vi "Tenney Main.vi"() -> ()   [LabVIEW 2023]
doc: "This template is for the Queued Message Handler design pattern.\n\nThe Event Handling Loop generates messages based on user interface actions.\n\nThe Message Handling Loop processes messages generated by the Event Handling Loop, or by other messages. The messages are string values, so new messages can be added easily to the Message Cases case structure in the Message Handling Loop. Each message cluster can also provide an optional value for Message Data, which is a variant that can be converted to whatever message-specific data is required."
uses:
  Drivers/Tidal Engineering/Type Definitions/Tenney Environmental Chamber Data.ctl
  controls/Tenney Temperature Limits.ctl
  Drivers/Viasala Indigo 520/Type Definitions/Viasala Indigo 520 Data.ctl
  Drivers/Tidal Engineering/Type Definitions/Tenney Chamber Status.ctl
  controls/Tenney UI Data.ctl
  support/Message Queue/Enqueue Message (Single).vi
  <vilib>/Utility/error.llb/Error Cluster From Error Code.vi
  <vilib>/ErrorRing/Error Ring.xnode
  support/Message Queue/Tenney Message Queue.lvlib
  support/User Event - Stop/Tenney User Event - Stop.lvlib
panel:
  in  "Tab Control":enum32{"Main", "Admin", "Debug Array"}(tab)
  in  "Chamber Status":T1
  in  "Set Status":bool
  in  "Set Temperature":bool
  in  "Set Humidity":bool
  in  "Set Frequency":bool
  in  "Setpoint Temperature (F)":dbl=67.5 min=32.0 max=135.0
  in  "Setpoint Humidity (%)":dbl=50.0 min=0.0 max=100.0
  in  "Setpoint Frequency (Hz)":dbl=10.0 min=5.0 max=60.0
  in  "Temperature Limits":T2={"Target Temperature Upper limit"=68.75, "Target Temperature Lower limit"=67.75, "Target Humidity Lower limit"=48.5, "Target Humidity Upper limit"=50.5, "Chamber Temperature Upper limit"=73.0, "Chamber Temperature Lower limit"=63.0, "Chamber Humidity Lower limit"=40.0, "Chamber Humidity Upper limit"=55.0, "Chamber Adjustment Increment (F)"=0.25, "Chamber Adjustment Interval (Minutes)"=10.0, "Chamber Adjustment Increment (%)"=0.25, "Chamber Adjustment Interval Fast (Minutes)"=10.0}
  in  "Update Temperature Limits":bool
  out "Tenney Data":T3
  out "Viasala Data Output":T4
  in  "Elapsed Time (Min)":dbl
  in  "Enable Auto Control":bool
  in  "Sample Rate (mS)":u32=10000
  in  "Viasala Loop Counter":i32
  in  "Viasala IP Address":string="10.2.0.39"
  in  "Tenney IP Address":string="10.2.0.248"
  in  "Debug":bool
  in  "Tenney Chamber Loop Counter":i32
  in  "Data Array":dbl[][](array[numeric])
  in  "Connect Viasala Counter":dbl
  in  "Connect Tenney Counter":dbl
  out "Main Array":string[](array[string])
  out "Tenney Array":string[](array[string])
  out "Viasala Array":string[](array[string])
  in  "Enable Arrays":bool
  in  "Exit":bool
  # "Tenney Chamber Manual Control"
  # "Data Output"
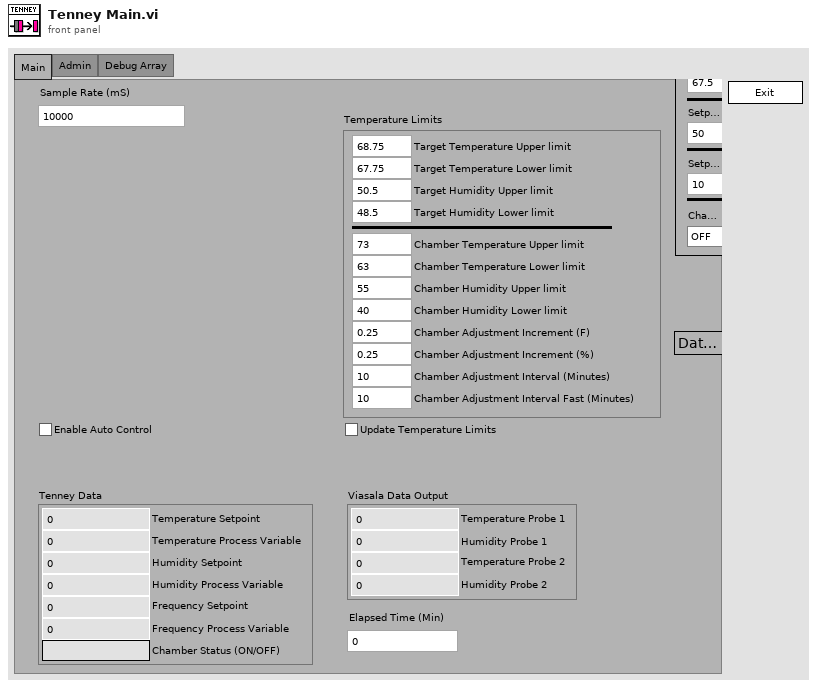
[diagram p1: front panel]
types:
  T1 = typedef "Tenney Chamber Status.ctl" = enum16{"OFF", "ON"}
  T2 = typedef "Tenney Temperature Limits.ctl" = cluster{"Target Temperature Upper limit":dbl, "Target Temperature Lower limit":dbl, "Target Humidity Lower limit":dbl, "Target Humidity Upper limit":dbl, "Chamber Temperature Upper limit":dbl, "Chamber Temperature Lower limit":dbl, "Chamber Humidity Lower limit":dbl, "Chamber Humidity Upper limit":dbl, "Chamber Adjustment Increment (F)":dbl, "Chamber Adjustment Interval (Minutes)":dbl, "Chamber Adjustment Increment (%)":dbl, "Chamber Adjustment Interval Fast (Minutes)":dbl}
  T3 = typedef "Tenney Environmental Chamber Data.ctl" = cluster{"Temperature Setpoint":dbl, "Temperature Process Variable":dbl, "Humidity Setpoint":dbl, "Humidity Process Variable":dbl, "Frequency Setpoint":dbl, "Frequency Process Variable":dbl, "Chamber Status (ON/OFF)":string}
  T4 = typedef "Viasala Indigo 520 Data.ctl" = cluster{"Temperature Probe 1":dbl, "Humidity Probe 1":dbl, "Temperature Probe 2":dbl, "Humidity Probe 2":dbl}
  T5 = typedef "Tenney UI Data.ctl" = cluster{"User Message":string, "Do Something Ref":refnum<vi>, "Do Something Else Ref":refnum<vi>, "Exit Button Ref":refnum<vi>}
  T6 = typedef "Tenney Message Queue.lvlib/All Message Queues.ctl" = cluster{"UI":refnum<queue>, "Tenney Chamber":refnum<queue>, "Viasala Humidity":refnum<queue>}
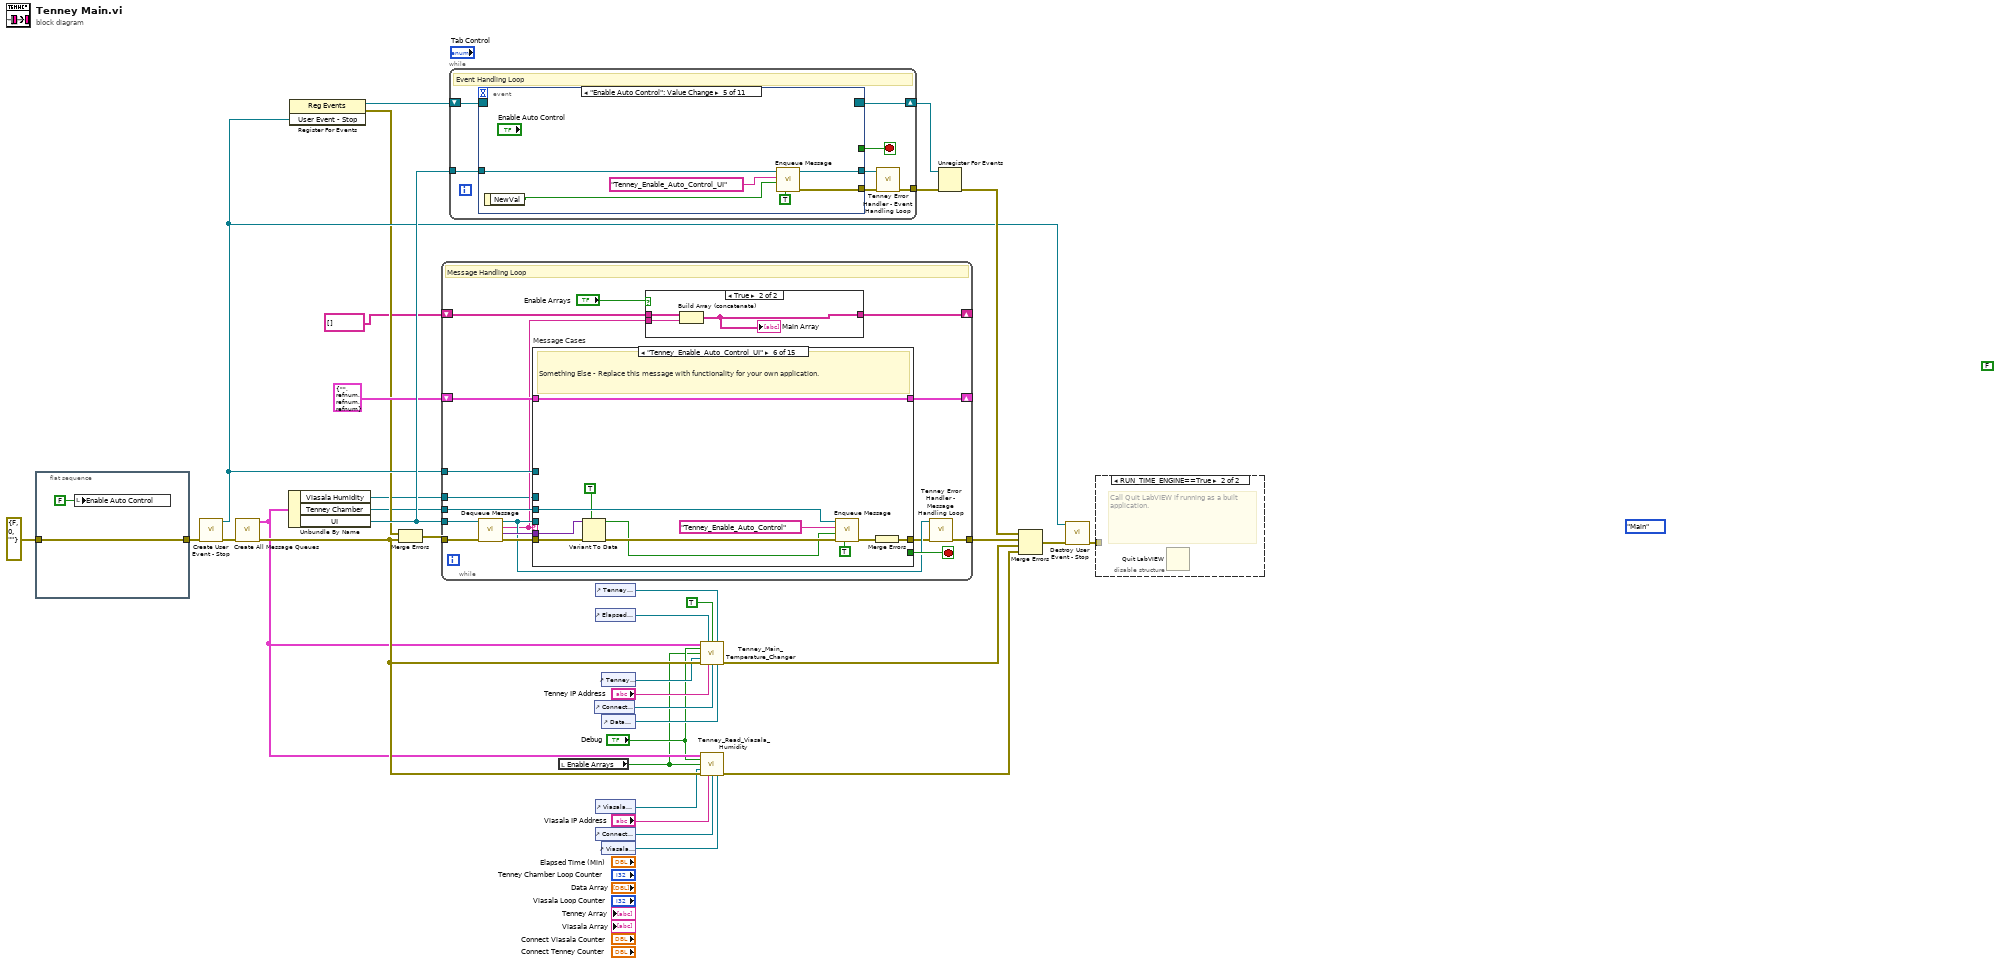
[diagram p0: block diagram]
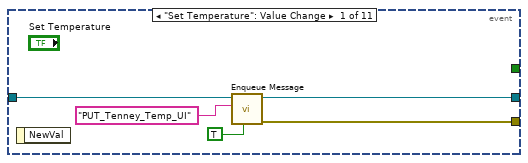
[diagram p3: hidden frame]
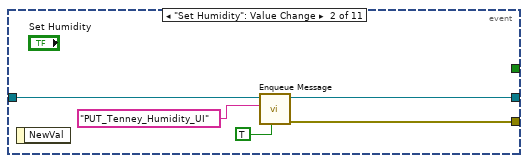
[diagram p4: hidden frame]
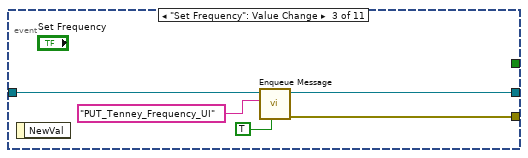
[diagram p5: hidden frame]
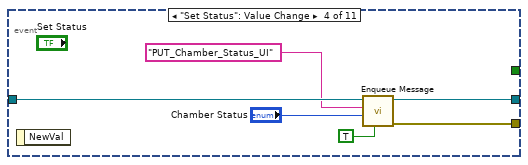
[diagram p6: hidden frame]
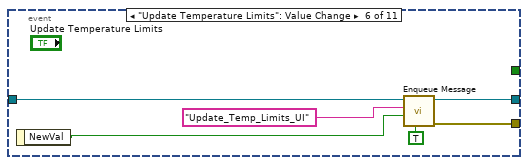
[diagram p7: hidden frame]
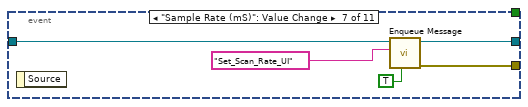
[diagram p8: hidden frame]
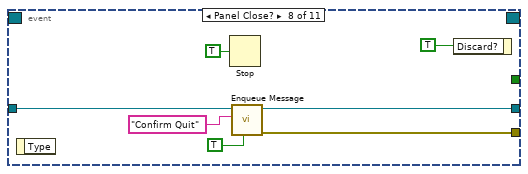
[diagram p9: hidden frame]
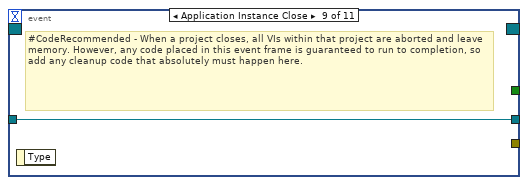
[diagram p10: hidden frame]
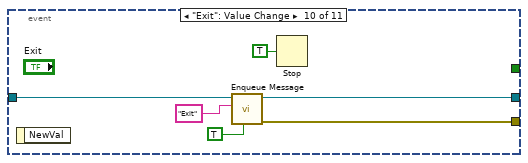
[diagram p11: hidden frame]
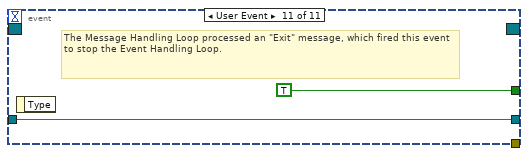
[diagram p12: hidden frame]
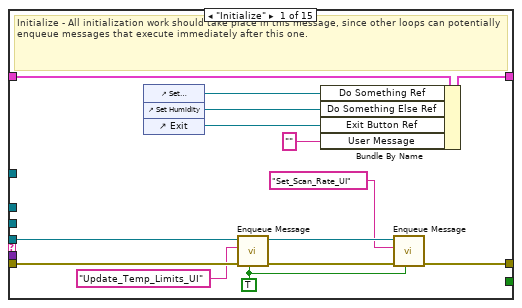
[diagram p14: hidden frame]
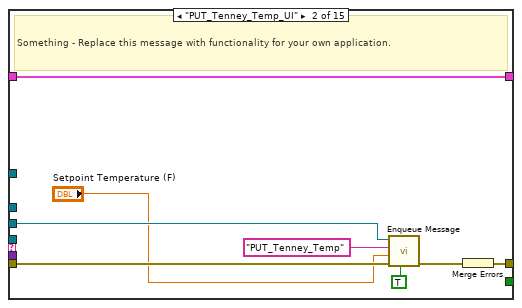
[diagram p15: hidden frame]
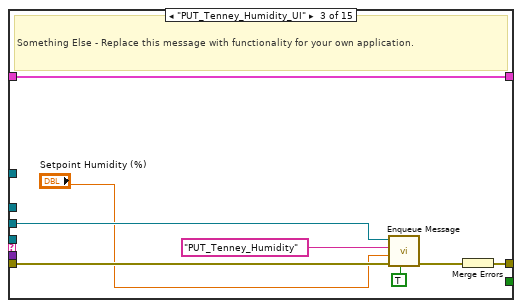
[diagram p16: hidden frame]
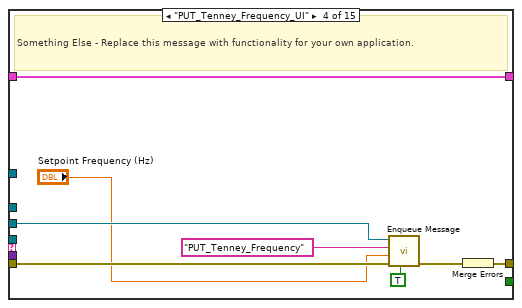
[diagram p17: hidden frame]
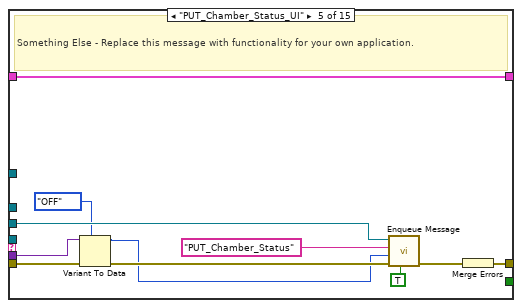
[diagram p18: hidden frame]
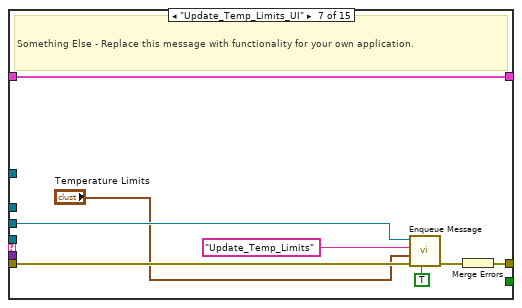
[diagram p19: hidden frame]
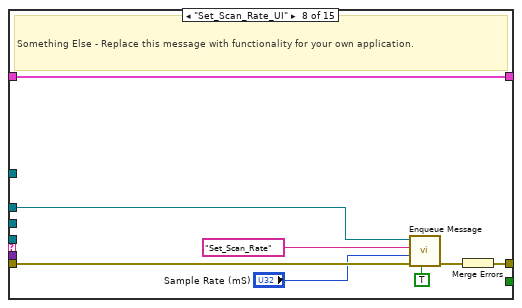
[diagram p20: hidden frame]
diagram:
  (unwired) FALSE ("Exit")
  (unwired) enum32{"Main", "Admin", "Debug Array"}."Main" ("Tab Control 8")
  n1 = flat-sequence {
    tunnel: errorcluster {"status"=FALSE, "code"=0, "source"=""} ("error in (no error)") -> [w37]
    tunnel: [w37] -> w18
    frame #0 {
      n2 = local write "Enable Auto Control"(FALSE ("Enable Auto Control")) -> ()
    }
  }
  n3 = call "Create User Event - Stop.vi"("error in (no error)"=w18) -> ("error out"=w33:errorcluster, "User Event - Stop"=w25:refnum<user-event>)  [unwired: 9 in]
  n4 = call "Create All Message Queues.vi"("error in (no error)"=w33) -> ("error out"=w17:errorcluster, "Message Queues out"=w15:T6)  [unwired: 9 in]
  n5 = Unbundle By Name(w15) -> ("Viasala Humidity"=w12:refnum<queue>, "Tenney Chamber"=w21:refnum<queue>, "UI"=w34:refnum<queue>)
  n6 = register-events(w25) -> (reference out=w26:refnum<event-registration>, error out=w23:errorcluster)  [unwired: 2 in]
  n7 = Merge Errors(w23, w17) -> (w24:errorcluster)
  n8 = while {
    tunnel: w34 -> [w47]
    shift-right: [w53] -> _
    shift-left: T5 {"User Message"="", "Do Something Ref"=refnum, "Do Something Else Ref"=refnum, "Exit Button Ref"=refnum} ("Data Cluster") -> [w54]
    tunnel: w25 -> [w51]
    tunnel: w24 -> [w50]
    tunnel: [w45] -> w35
    tunnel: w21 -> [w43]
    shift-right: [w41] -> _
    shift-left: string[] [] -> [w42]
    tunnel: w12 -> [w39]
    stop <- w52 stop-if-true
    # "Message Handling Loop"
    n9 = call "Dequeue Message.vi"("error in (no error)"=w50, "Message Queue"=w47) -> ("error out"=w49:errorcluster, "Message Data"=w48:variant, "Message"=w40:string, "dup Message Queue"=w46:refnum<queue>)  [unwired: 6 in]
    n10 = case "Message Cases" shown="\"Tenney_Enable_Auto_Control_UI\"" w40 {
      selector: w40 -> [_ _ _ _ _ _ _ _ _ _ _ _ _ _ w183]
      tunnel: w46 -> [w66 _ _ _ _ _ _ _ _ _ _ w158 _ w182 _]
      tunnel: w49 -> [w65 w78 w86 w94 w101 w112 w120 w129 w139 w146 w155 w162 w165 w176 _]
      tunnel: [w62 w79 w87 w95 w106 w117 w125 w133 w140 w147 w149 w160 w163 w179 w184] -> w44
      tunnel: w54 -> [w72 w80 w88 w96 w107 w118 w126 w134 w141 w148 w154 w161 w164 w181 w185]
      tunnel: [w71 w80 w88 w96 w107 w118 w126 w134 w141 w148 w154 w161 w164 w181 w185] -> w53
      tunnel: [_ _ _ _ _ _ _ _ _ _ _ _ _ TRUE _] -> w52
      tunnel: w48 -> [_ _ _ _ w99 w110 _ _ w138 w145 w153 _ _ w173 _]
      tunnel: w51 -> [_ _ _ _ _ _ _ _ _ _ _ _ _ w178 _]
      tunnel: w43 -> [_ w75 w83 w91 w103 w114 w122 _ _ _ _ _ _ w171 _]
      tunnel: w39 -> [_ _ _ _ _ _ _ w127 _ _ _ _ _ w168 _]
      frame "Initialize" {
        w60 = TRUE ("Priority Message? (F)")
        # "Initialize - All initialization work should take place in this message, since other loops can potentially enqueue messages that execute immediately after this one."
        n11 = control-ref of="Set Temperature"() -> (w70:refnum<vi>)
        n12 = control-ref of="Set Humidity"() -> (w69:refnum<vi>)
        n13 = control-ref of="Exit"() -> (w68:refnum<vi>)
        n14 = call-poly "Enqueue Message.vi"("Priority Message? (F)"=w60, "error in (no error)"=w65, "Message"="Update_Temp_Limits_UI", "Message Queue"=w66) -> ("error out"=w63:errorcluster, "dup Message Queue"=w61:refnum<queue>)  [unwired: 6 in]
        n15 = Bundle By Name(cluster=w72, "Do Something Ref"=w70, "Do Something Else Ref"=w69, "Exit Button Ref"=w68, "User Message"="" ("Initial Message")) -> (w71:T5)
        n16 = call-poly "Enqueue Message.vi"("Priority Message? (F)"=w60, "error in (no error)"=w63, "Message"="Set_Scan_Rate_UI", "Message Queue"=w61) -> ("error out"=w62:errorcluster)  [unwired: 6 in, 1 out]
      }
      frame "PUT_Tenney_Temp_UI" {
        # "Something - Replace this message with functionality for your own application."
        n17 = call-poly "Enqueue Message.vi"("Priority Message? (F)"=TRUE, "error in (no error)"=w78, "Message Data"="Setpoint Temperature (F)", "Message"="PUT_Tenney_Temp", "Message Queue"=w75) -> ("error out"=w77:errorcluster)  [unwired: 5 in, 1 out]
        n18 = Merge Errors(w77) -> (w79:errorcluster)
      }
      frame "PUT_Tenney_Humidity_UI" {
        # "Something Else - Replace this message with functionality for your own application."
        n19 = call-poly "Enqueue Message.vi"("Priority Message? (F)"=TRUE, "error in (no error)"=w86, "Message Data"="Setpoint Humidity (%)", "Message"="PUT_Tenney_Humidity", "Message Queue"=w83) -> ("error out"=w85:errorcluster)  [unwired: 5 in, 1 out]
        n20 = Merge Errors(w85) -> (w87:errorcluster)
      }
      frame "PUT_Tenney_Frequency_UI" {
        # "Something Else - Replace this message with functionality for your own application."
        n21 = call-poly "Enqueue Message.vi"("Priority Message? (F)"=TRUE, "error in (no error)"=w94, "Message Data"="Setpoint Frequency (Hz)", "Message"="PUT_Tenney_Frequency", "Message Queue"=w91) -> ("error out"=w93:errorcluster)  [unwired: 5 in, 1 out]
        n22 = Merge Errors(w93) -> (w95:errorcluster)
      }
      frame "PUT_Chamber_Status_UI" {
        # "Something Else - Replace this message with functionality for your own application."
        n23 = Variant To Data(error in=w101, type=Tenney_Chamber_Status."OFF" ("Chamber Status"), Variant=w99) -> (data=w97:T1, error out=w100:errorcluster)
        n24 = call-poly "Enqueue Message.vi"("Priority Message? (F)"=TRUE, "error in (no error)"=w100, "Message Data"=w97, "Message"="PUT_Chamber_Status", "Message Queue"=w103) -> ("error out"=w105:errorcluster)  [unwired: 5 in, 1 out]
        n25 = Merge Errors(w105) -> (w106:errorcluster)
      }
      frame "Tenney_Enable_Auto_Control_UI" {
        # "Something Else - Replace this message with functionality for your own application."
        n26 = Variant To Data(error in=w112, type=TRUE, Variant=w110) -> (data=w109:bool, error out=w111:errorcluster)
        n27 = call-poly "Enqueue Message.vi"("Priority Message? (F)"=TRUE, "error in (no error)"=w111, "Message Data"=w109, "Message"="Tenney_Enable_Auto_Control", "Message Queue"=w114) -> ("error out"=w116:errorcluster)  [unwired: 5 in, 1 out]
        n28 = Merge Errors(w116) -> (w117:errorcluster)
      }
      frame "Update_Temp_Limits_UI" {
        # "Something Else - Replace this message with functionality for your own application."
        n29 = call-poly "Enqueue Message.vi"("Priority Message? (F)"=TRUE, "error in (no error)"=w120, "Message Data"="Temperature Limits", "Message"="Update_Temp_Limits", "Message Queue"=w122) -> ("error out"=w124:errorcluster)  [unwired: 5 in, 1 out]
        n30 = Merge Errors(w124) -> (w125:errorcluster)
      }
      frame "Set_Scan_Rate_UI" {
        # "Something Else - Replace this message with functionality for your own application."
        n31 = call-poly "Enqueue Message.vi"("Priority Message? (F)"=TRUE, "error in (no error)"=w129, "Message Data"="Sample Rate (mS)", "Message"="Set_Scan_Rate", "Message Queue"=w127) -> ("error out"=w132:errorcluster)  [unwired: 5 in, 1 out]
        n32 = Merge Errors(w132) -> (w133:errorcluster)
      }
      frame "DisplayValuesFromTenney" {
        # "Update Display - Convert the message data to a string to display in the Data Display indicator."
        n33 = Variant To Data(error in=w139, type=T3 {"Temperature Setpoint"=0.0, "Temperature Process Variable"=0.0, "Humidity Setpoint"=0.0, "Humidity Process Variable"=0.0, "Frequency Setpoint"=0.0, "Frequency Process Variable"=0.0, "Chamber Status (ON/OFF)"=""} ("Tenney Environmental Chamber Data"), Variant=w138) -> (data=→"Tenney Data":T3, error out=w137:errorcluster)
        n34 = Merge Errors(w137) -> (w140:errorcluster)
      }
      frame "DisplayValuesFromViasala" {
        # "Update Display - Convert the message data to a string to display in the Data Display indicator."
        n35 = Variant To Data(error in=w146, type=T4 {"Temperature Probe 1"=0.0, "Humidity Probe 1"=0.0, "Temperature Probe 2"=0.0, "Humidity Probe 2"=0.0} ("Viasala Data Output"), Variant=w145) -> (data=→"Viasala Data Output":T4, error out=w144:errorcluster)
        n36 = Merge Errors(w144) -> (w147:errorcluster)
      }
      frame "Error" {
        # "Error - Display an error dialog. This message is sent by the \"Error Handler\" VIs at the end of other loops in this application."
        n37 = Variant To Data(error in=w155, type=errorcluster {"status"=FALSE, "code"=0, "source"=""} ("error constant"), Variant=w153) -> (data=w151:errorcluster, error out=w150:errorcluster)
        n38 = call <vilib>:"Simple Error Handler.vi"("error in (no error)"=w151) -> ()  [unwired: 4 in, 5 out]
        n39 = Merge Errors(w150) -> (w149:errorcluster)
      }
      frame "Confirm Quit" {
        # "Confirm Quit - Message that can confirm whether or not the user wants to exit the application."
        n40 = call-poly "Enqueue Message.vi"("Priority Message? (F)"=TRUE, "error in (no error)"=w162, "Message"="Exit", "Message Queue"=w158) -> ("error out"=w159:errorcluster)  [unwired: 6 in, 1 out]
        n41 = Merge Errors(w159) -> (w160:errorcluster)
      }
      frame "---Copy This Frame---" {
        # "Duplicate this frame when creating new messages.  Change this comment in the duplicated frame to describe this message."
        n42 = Merge Errors(w165) -> (w163:errorcluster)
      }
      frame "Exit" {
        w166 = TRUE ("Priority Message? (F)")
        w167 = "Exit" ("Message")
        # "Exit - Exit the application."
        n43 = Variant To Data(type=errorcluster {"status"=FALSE, "code"=0, "source"=""} ("error constant"), Variant=w173) -> (data=w174:errorcluster)  [unwired: 1 in, 1 out]
        n44 = call <vilib>:"Simple Error Handler.vi"("error in (no error)"=w174) -> ()  [unwired: 4 in, 5 out]
        n45 = call "Fire User Event - Stop.vi"("User Event - Stop"=w178) -> ("error out"=w177:errorcluster)  [unwired: 10 in]
        n46 = Release Queue(queue=w182, error in (no error)=w176) -> (error out=w172:errorcluster)  [unwired: 1 in, 2 out]
        n47 = call-poly "Enqueue Message.vi"("Priority Message? (F)"=w166, "error in (no error)"=w172, "Message"=w167, "Message Queue"=w171) -> ("error out"=w170:errorcluster)  [unwired: 6 in, 1 out]
        n48 = call-poly "Enqueue Message.vi"("Priority Message? (F)"=w166, "error in (no error)"=w170, "Message"=w167, "Message Queue"=w168) -> ("error out"=w169:errorcluster)  [unwired: 6 in, 1 out]
        n49 = Merge Errors(w177, w169) -> (w179:errorcluster)
      }
      frame Default {
        # "'Default' case only runs if there is a message that isn't defined in any of the other cases.  Output a programming error."
        n50 = xnode "Error Ring"("parameter 0"=w183) -> ("error out"=w184:errorcluster)
      }
    }
    n51 = case shown="True" "Enable Arrays" {
      tunnel: w42 -> [w55 w58]
      tunnel: [w55 w57] -> w41
      tunnel: w40 -> [_ w56]
      frame False {
      }
      frame True {
        n52 = Build Array (concatenate)(w58, w56) -> (w57:string[])
        "Main Array" <- w57
      }
    }
    n53 = call "Tenney Error Handler - Message Handling Loop.vi"("error in (no error)"=w44, "Message Queue"=w46) -> ("dup error in"=w45:errorcluster)  [unwired: 8 in, 1 out]
  }
  n54 = while {
    tunnel: w34 -> [w199]
    shift-right: [w197] -> w30
    shift-left: w26 -> [w198]
    tunnel: [w193] -> w27
    stop <- w195 stop-if-true
    # "Event Handling Loop"
    n55 = event shown="[4] \"Enable Auto Control\": Value Change" {
      selector: w198 -> [_ _ _ _ _ _ _ _ _ _ _]
      dyn-events: [_ _ _ _ _ _ _ _ _ _ _] -> w197
      timeout: _ -> [_ _ _ _ _ _ _ _ _ _ _]
      tunnel: [_ _ _ _ _ _ _ _ _ _ TRUE ("Discard?")] -> w195
      tunnel: w199 -> [w204 w209 w214 w220 w226 w232 w235 w243 w245 w251 w253]
      tunnel: [w201 w206 w211 w217 w223 w229 w233 w242 _ w250 _] -> w196
      tunnel: [w203 w208 w213 w219 w225 w231 w234 w241 w245 w249 w253] -> w194
      event "Set Temperature": Value Change {
        n56 = event-data() -> ()  [unwired: 1 in, 1 out]
        n57 = call-poly "Enqueue Message.vi"("Priority Message? (F)"=TRUE, "Message"="PUT_Tenney_Temp_UI", "Message Queue"=w204) -> ("error out"=w201:errorcluster, "dup Message Queue"=w203:refnum<queue>)  [unwired: 7 in]
      }
      event "Set Humidity": Value Change {
        n58 = event-data() -> ()  [unwired: 1 in, 1 out]
        n59 = call-poly "Enqueue Message.vi"("Priority Message? (F)"=TRUE, "Message"="PUT_Tenney_Humidity_UI", "Message Queue"=w209) -> ("error out"=w206:errorcluster, "dup Message Queue"=w208:refnum<queue>)  [unwired: 7 in]
      }
      event "Set Frequency": Value Change {
        n60 = event-data() -> ()  [unwired: 1 in, 1 out]
        n61 = call-poly "Enqueue Message.vi"("Priority Message? (F)"=TRUE, "Message"="PUT_Tenney_Frequency_UI", "Message Queue"=w214) -> ("error out"=w211:errorcluster, "dup Message Queue"=w213:refnum<queue>)  [unwired: 7 in]
      }
      event "Set Status": Value Change {
        n62 = event-data() -> ()  [unwired: 1 in, 1 out]
        n63 = call-poly "Enqueue Message.vi"("Priority Message? (F)"=TRUE, "Message Data"="Chamber Status", "Message"="PUT_Chamber_Status_UI", "Message Queue"=w220) -> ("error out"=w217:errorcluster, "dup Message Queue"=w219:refnum<queue>)  [unwired: 6 in]
      }
      event "Enable Auto Control": Value Change {
        n64 = event-data() -> ("NewVal"=w222:bool)  [unwired: 1 in]
        n65 = call-poly "Enqueue Message.vi"("Priority Message? (F)"=TRUE, "Message Data"=w222, "Message"="Tenney_Enable_Auto_Control_UI", "Message Queue"=w226) -> ("error out"=w223:errorcluster, "dup Message Queue"=w225:refnum<queue>)  [unwired: 6 in]
      }
      event "Update Temperature Limits": Value Change {
        n66 = event-data() -> ("NewVal"=w228:bool)  [unwired: 1 in]
        n67 = call-poly "Enqueue Message.vi"("Priority Message? (F)"=TRUE, "Message Data"=w228, "Message"="Update_Temp_Limits_UI", "Message Queue"=w232) -> ("error out"=w229:errorcluster, "dup Message Queue"=w231:refnum<queue>)  [unwired: 6 in]
      }
      event "Sample Rate (mS)": Value Change {
        n68 = event-data() -> ()  [unwired: 1 in, 1 out]
        n69 = call-poly "Enqueue Message.vi"("Priority Message? (F)"=TRUE, "Message"="Set_Scan_Rate_UI", "Message Queue"=w235) -> ("error out"=w233:errorcluster, "dup Message Queue"=w234:refnum<queue>)  [unwired: 7 in]
      }
      event Panel Close? {
        n70 = event-data() -> ()  [unwired: 1 in, 1 out]
        n71 = Stop(stop? (T)=TRUE) -> ()
        n72 = call-poly "Enqueue Message.vi"("Priority Message? (F)"=TRUE, "Message"="Confirm Quit", "Message Queue"=w243) -> ("error out"=w242:errorcluster, "dup Message Queue"=w241:refnum<queue>)  [unwired: 7 in]
        n73 = event-data("Discard?"=TRUE) -> ()  [unwired: 1 in, 1 out]
      }
      event Application Instance Close {
        # "#CodeRecommended - When a project closes, all VIs within that project are aborted and leave memory. However, any code placed in this event frame is guaranteed to run to completion, so add any cleanup code that absolutely must happen here."
        n74 = event-data() -> ()  [unwired: 1 in, 1 out]
      }
      event "Exit": Value Change {
        n75 = event-data() -> ()  [unwired: 1 in, 1 out]
        n76 = call-poly "Enqueue Message.vi"("Priority Message? (F)"=TRUE, "Message"="Exit", "Message Queue"=w251) -> ("error out"=w250:errorcluster, "dup Message Queue"=w249:refnum<queue>)  [unwired: 7 in]
        n77 = Stop(stop? (T)=TRUE) -> ()
      }
      event User Event {
        # "The Message Handling Loop processed an \"Exit\" message, which fired this event to stop the Event Handling Loop."
        n78 = event-data() -> ()  [unwired: 1 in, 1 out]
      }
    }
    n79 = call "Tenney Error Handler - Event Handling Loop.vi"("error in (no error)"=w196, "Message Queue"=w194) -> ("dup error in"=w193:errorcluster)  [unwired: 8 in, 1 out]
  }
  n80 = local read "Enable Arrays"() -> (w2:bool)
  n81 = control-ref of="Connect Tenney Counter"() -> (w4:refnum<vi>)
  n82 = control-ref of="Tenney Chamber Loop Counter"() -> (w10:refnum<vi>)
  n83 = control-ref of="Elapsed Time (Min)"() -> (w11:refnum<vi>)
  n84 = control-ref of="Viasala Loop Counter"() -> (w8:refnum<vi>)
  n85 = control-ref of="Connect Viasala Counter"() -> (w5:refnum<vi>)
  n86 = control-ref of="Tenney Array"() -> (w7:refnum<vi>)
  n87 = control-ref of="Data Array"() -> (w9:refnum<vi>)
  n88 = control-ref of="Viasala Array"() -> (w6:refnum<vi>)
  n89 = call "Tenney_Main_Temperature_Changer.vi"("Message Queues out"=w15, "Elapsed Time (min) Ref"=w11, "Disable Tenney"=TRUE, "Loop Count Ref"=w10, "Debug"="Debug", "Enable Arrays"=w2, "Tenney Array"=w7, "error in"=w17, "Tenney IP Address"="Tenney IP Address", "Connect Tenney Ref"=w4, "Data Array"=w9) -> ("error out"=w22:errorcluster)  [unwired: 4 in]
  n90 = call "Tenney_Read_Viasala_Humidity.vi"("Message Queues out"=w15, "Debug"="Debug", "Enable Arrays"=w2, "Loop Count Ref"=w8, "error in"=w17, "Viasala IP Address"="Viasala IP Address", "Connect Viasala Ref"=w5, "Viasala Array"=w6) -> ("error out"=w16:errorcluster)  [unwired: 7 in]
  n91 = Unregister For Events(event registration refnum=w30, error in=w27) -> (error out=w31:errorcluster)
  n92 = Merge Errors(w31, w35, w22, w16) -> (w32:errorcluster)
  n93 = call "Destroy User Event - Stop.vi"("error in (no error)"=w32, "User Event - Stop"=w25) -> ("error out"=w28:errorcluster)  [unwired: 9 in]
  n94 = disable-structure shown="RUN_TIME_ENGINE==True" {
    disable-tunnel: w28 -> [_ _]
    frame condition #0 (active) {
    }
    frame condition #1 {
      # "Call Quit LabVIEW if running as a built application."
      n95 = Quit LabVIEW() -> ()  [unwired: 1 in]
    }
  }
